vi "Set Wheel Position by Index.vi"(8 "error in (no error)":errorcluster, 9 "active wheel indexes in":i32[](array[numeric]), 10 "position":dbl[](array[numeric]), 11 "steering frame ref in":refnum<data-value>) -> (0 "error out":errorcluster, 3 "steering frame ref out":refnum<data-value>)   [LabVIEW 2017, in "NI_Robotics_Configure Steering Frame.lvlib"]
uses:
  <vilib>/robotics/Dialog/Configure Steering Frame/NI_Robotics_Configure Steering Frame.lvlib
  <vilib>/robotics/Steering/Steering Frame/NI_Robotics_Steering Frame.lvclass
  <vilib>/robotics/Steering/Steering Frame/Reposition Single Wheel on Steering Frame.vi
  <vilib>/Utility/AngleManip/Degrees to Radians (Scalar DBL).vi
  <vilib>/Utility/AngleManip/NI_AngleManipulation.lvlib
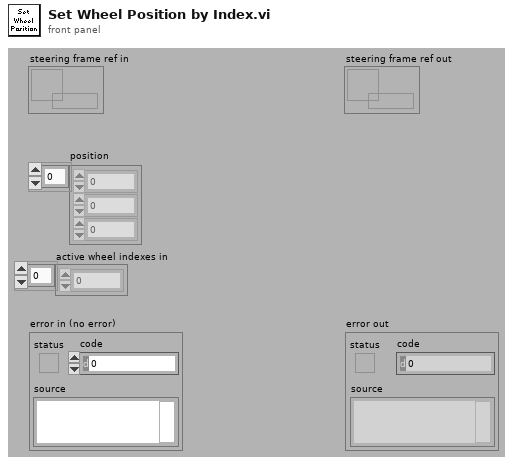
[diagram p1: front panel]
types:
  T1 = typedef "NI_Robotics_Configure Steering Frame.lvlib/Angle Mode.ctl" = u16
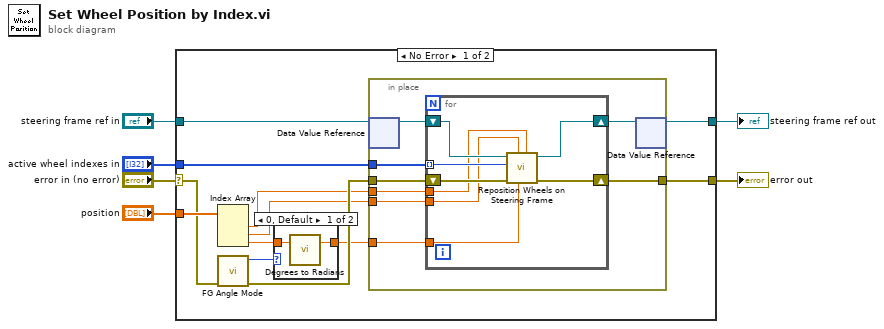
[diagram p0: block diagram]
diagram:
  n1 = case shown="No Error" "error in (no error)" {
    selector: "error in (no error)" -> [w12 w39]
    tunnel: [w18 w39] -> w5
    tunnel: "position" -> [w13 _]
    tunnel: "steering frame ref in" -> [w17 w38]
    tunnel: "active wheel indexes in" -> [w7 _]
    tunnel: [w16 w38] -> w1
    frame No Error {
      n2 = Index Array(array=w13) -> (element #1=w9:dbl, element #2=w8:dbl, element #3=w15:dbl)  [unwired: 3 in]
      n3 = call <vilib>:"FG Angle Mode.vi"("error in (no error)"=w12) -> ("error out"=w11:errorcluster, "angle mode out"=w14:T1)  [unwired: 9 in]
      n4 = case shown="0, Default" w14 {
        tunnel: w15 -> [w20 w21]
        tunnel: [w19 w21] -> w10
        frame 0, Default {
          n5 = call-poly <vilib>:"Degrees to Radians.vi"("angle (deg)"=w20) -> ("angle (rad)"=w19:dbl)  [unwired: 2 in]
        }
        frame 1 {
        }
      }
      n6 = in-place {
        in-place-border: [w27] -> w18
        in-place-border: w7 -> [w26]
        in-place-border: w11 -> [w25]
        in-place-border: w10 -> [w22]
        in-place-border: w9 -> [w24]
        in-place-border: w8 -> [w23]
        n7 = in-place-dvr #1(w17) -> (w29:refnum<class "NI_Robotics_Steering Frame.lvclass">)  [unwired: 1 out]
        n8 = for {
          tunnel: w26 -> [w34] mode=indexing
          tunnel: w24 -> [w32]
          tunnel: w23 -> [w31]
          tunnel: w22 -> [w30]
          shift-right: [w36] -> w28
          shift-left: w29 -> [w37]
          shift-right: [w35] -> w27
          shift-left: w25 -> [w33]
          n9 = call-poly <vilib>:"Reposition Wheels on Steering Frame.vi"("x position"=w32, "frame angle (rad)"=w30, "y position"=w31, "error in (no error)"=w33, "wheel index"=w34, "steering frame in"=w37) -> ("error out"=w35:errorcluster, "steering frame out"=w36:refnum<class "NI_Robotics_Steering Frame.lvclass">)  [unwired: 3 in, 1 out]
        }
        n10 = in-place-dvr #1(w28) -> (w16:refnum<data-value>)  [unwired: 1 out]
      }
    }
    frame Error {
    }
  }
  "error out" <- w5
  "steering frame ref out" <- w1
